vi "Main.vi"() -> ()   [LabVIEW 2021]
doc: "The myRIO Project template acquires acceleration data from the onboard accelerometer and displays the changes of acceleration values in a waveform chart."
uses:
  <vilib>/myRIO/Instrument Drivers/Onboard IO/AI/typedefs/AI Reference.ctl
  <vilib>/myRIO/Common/Instrument Driver Framework/Utilities/typedefs/myRIO Generic Hardware Reference.ctl
  <vilib>/myRIO/Common/Instrument Driver Framework/Utilities/typedefs/Hardware Version Enum.ctl
  <vilib>/myRIO/Common/Instrument Driver Framework/Utilities/typedefs/myRIO v1.0 Reference.ctl
  <vilib>/myRIO/Common/Instrument Driver Framework/Utilities/typedefs/Generic FPGA Reference.ctl
  <vilib>/myRIO/Common/Instrument Driver Framework/myRIO v1.0/AI/typedefs/AI Channels List.ctl
  <vilib>/myRIO/Common/Instrument Driver Framework/myRIO v1.0/AI/typedefs/AI Channels Enum.ctl
  <vilib>/myRIO/Common/Instrument Driver Framework/Utilities/typedefs/Analog Scaling Constants List.ctl
  <vilib>/myRIO/Common/Instrument Driver Framework/Utilities/typedefs/Analog Scaling Constants.ctl
  <vilib>/userDefined/High Color/nirio_resource_hc.ctl
  <vilib>/myRIO/Instrument Drivers/Onboard IO/DIO/typedefs/DIO Reference.ctl
  <vilib>/myRIO/Common/Instrument Driver Framework/myRIO v1.0/DIO/typedefs/DIO Channels List.ctl
  <vilib>/myRIO/Common/Instrument Driver Framework/myRIO v1.0/DIO/typedefs/DIO Channels Enum.ctl
  <vilib>/myRIO/Instrument Drivers/Onboard IO/PWM/typedefs/PWM Reference.ctl
  <vilib>/myRIO/Common/Instrument Driver Framework/myRIO v1.0/PWM/typedefs/PWM Channels Enum.ctl
  <vilib>/myRIO/Instrument Drivers/Onboard IO/PWM/typedefs/PWM Configuration.ctl
  <vilib>/myRIO/Common/Instrument Driver Framework/Utilities/vis/Is FPGA Ref Available.vi
  <vilib>/myRIO/Common/Instrument Driver Framework/myRIO v1.0/AI/vis/myRIO v1.1 Open AI.vi
  <vilib>/myRIO/Instrument Drivers/Onboard IO/AI/vis/Read.vi
  <vilib>/myRIO/Common/Instrument Driver Framework/myRIO v1.0/DIO/vis/myRIO v1.1 Open DIO.vi
  <vilib>/myRIO/Instrument Drivers/Onboard IO/DIO/vis/Write.vi
  <vilib>/myRIO/Common/Instrument Driver Framework/myRIO v1.0/PWM/vis/myRIO v1.1 Open PWM.vi
  <vilib>/myRIO/Instrument Drivers/Onboard IO/PWM/vis/Set Duty Cycle and Frequency.vi
  <vilib>/myRIO/Common/Instrument Driver Framework/Utilities/vis/Validate Channels.vi
  <vilib>/myRIO/Common/Instrument Driver Framework/myRIO v1.0/AI/vis/myRIO v1.0 Reserve AI.vi
  <vilib>/myRIO/Common/Instrument Driver Framework/myRIO v1.0/DIO/vis/myRIO v1.0 Reserve DIO.vi
  <vilib>/myRIO/Common/Instrument Driver Framework/myRIO v1.0/PWM/vis/myRIO v1.0 Reserve PWM.vi
  <vilib>/myRIO/Common/Instrument Driver Framework/myRIO v1.0/AI/vis/myRIO v1.0 Build MUX Configuration AI.vi
  <vilib>/myRIO/Common/Instrument Driver Framework/myRIO v1.0/Resource Manager/vis/myRIO v1.0 Reserve Channel List.vi
  <vilib>/myRIO/Common/Instrument Driver Framework/myRIO v1.0/DIO/vis/myRIO v1.0 Build MUX Configuration DIO.vi
  <vilib>/myRIO/Common/Instrument Driver Framework/myRIO v1.0/PWM/vis/myRIO v1.0 Build MUX Configuration PWM.vi
  <vilib>/myRIO/Common/Instrument Driver Framework/myRIO v1.0/Resource Manager/vis/myRIO v1.0 Reserve Channel.vi
  <vilib>/myRIO/Common/Instrument Driver Framework/myRIO v1.0/Resource Manager/vis/myRIO v1.0 Unreserve Channel.vi
  <vilib>/myRIO/Common/Instrument Driver Framework/myRIO v1.0/Resource Manager/vis/myRIO v1.0 Create Configuration List.vi
  <vilib>/myRIO/Common/Instrument Driver Framework/myRIO v1.0/Resource Manager/vis/myRIO v1.0 Build Mutex Name.vi
  <vilib>/Utility/VariantDataType/GetNumericInfo.vi
  <vilib>/Utility/error.llb/Error Cluster From Error Code.vi
  <vilib>/myRIO/Common/Instrument Driver Framework/myRIO v1.0/myRIO v1.1 Open.vi
  <vilib>/myRIO/Common/Instrument Driver Framework/myRIO v1.0/AI/vis/myRIO v1.0 Get Scaling Constants AI.vi
  <vilib>/myRIO/Common/Instrument Driver Framework/Utilities/vis/IO Manager.vi
  <vilib>/myRIO/Common/Instrument Driver Framework/Utilities/vis/Configuration Manager.vi
  <vilib>/myRIO/Common/Instrument Driver Framework/myRIO v1.0/myRIO v1.0 Close.vi
  <vilib>/myRIO/Common/Instrument Driver Framework/myRIO v1.0/AI/vis/myRIO v1.0 Read AI.vi
  <vilib>/myRIO/Common/Instrument Driver Framework/myRIO v1.0/Resource Manager/vis/myRIO v1.0 Configure IO.vi
  <vilib>/myRIO/Common/Instrument Driver Framework/myRIO v1.0/DIO/vis/myRIO v1.0 Write DIO.vi
  <vilib>/addons/control/pid/pid.llb/PID (DBL).vi
  <vilib>/myRIO/Common/Instrument Driver Framework/myRIO v1.0/PWM/vis/myRIO v1.0 Write PWM.vi
  <vilib>/myRIO/Express VI/Onboard IO/AI/AI Express VI.xnode
  <vilib>/myRIO/Instrument Drivers/Onboard IO/AI/vis/myRIO AI Open.xnode
  <vilib>/myRIO/Express VI/Onboard IO/DO/DO Express VI.xnode
  <vilib>/myRIO/Instrument Drivers/Onboard IO/DIO/vis/myRIO DIO Open.xnode
  <vilib>/myRIO/Express VI/Onboard IO/PWM/PWM Express VI.xnode
  <vilib>/myRIO/Instrument Drivers/Onboard IO/PWM/vis/myRIO PWM Open.xnode
  <vilib>/myRIO/Instrument Drivers/Onboard IO/AI/AI.lvlib
  <vilib>/myRIO/Instrument Drivers/Onboard IO/DIO/DIO.lvlib
  <vilib>/addons/control/pid/NI_PID_pid.lvlib
  <vilib>/myRIO/Instrument Drivers/Onboard IO/PWM/PWM.lvlib
panel:
  out "Array Index":dbl
  out "Target Angle Reached":bool
  in  "Drop-Off Angle":dbl=90.0
  in  "Complete Stop Angle":dbl=45.0
  out "Target Angle":dbl
  out "Drop-Off Position":dbl
  out "Complete Stop Position":dbl
  in  "PID Gains":T1={"Proportional Gain, Kc"=0.5, "Integral Time, ti"=0.1, "Derivative Time, td"=0.1}
  out "Run Motor PWM":dbl
  in  "Manual Mode switch":bool
  in  "DIO4":bool
  in  "DIO5":bool
  in  "DIO6":bool
  in  "DIO7":bool
  out "Upper limit":bool
  out "Lower Limit":bool
  in  "Home Position":dbl=250.0
  out "Angle":dbl
  out "AI3":dbl
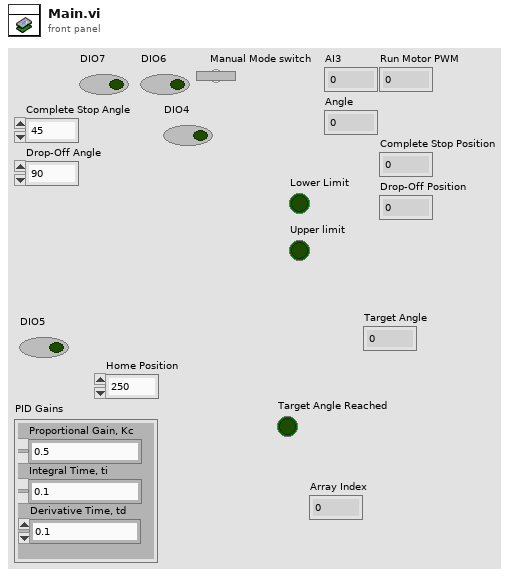
[diagram p1: front panel]
types:
  T1 = cluster{"Proportional Gain, Kc":dbl, "Integral Time, ti":dbl, "Derivative Time, td":dbl}
  T2 = typedef "DIO.lvlib/DIO Reference.ctl" = cluster{"myRIO Reference":T3, "DIO Channels List":T7}
  T3 = typedef "myRIO Generic Hardware Reference.ctl" = cluster{"myRIO Model":T4, "myRIO Hardware Reference":T5}
  T4 = typedef "Hardware Version Enum.ctl" = enum16{"Unknown", "myRIO-1900", "myRIO-1950", "roboRIO", "NI ELVIS RIO CM", "ELVIS III"}
  T5 = typedef "myRIO v1.0 Reference.ctl" = cluster{"Generic FPGA Reference":T6, "Allow multiple opens":bool}
  T6 = typedef "Generic FPGA Reference.ctl" = refnum<k20>
  T7 = typedef "DIO Channels List.ctl" = T8[]
  T8 = typedef "DIO Channels Enum.ctl" = enum16{"Not Connected", "C/DIO0", "C/DIO1", "C/DIO2", "C/DIO3", "C/DIO4", "C/DIO5", "C/DIO6", "C/DIO7", "A/DIO0", "A/DIO1", "A/DIO2", "A/DIO3", "A/DIO4", "A/DIO5", "A/DIO6", "A/DIO7", "A/DIO8", "A/DIO9", "A/DIO10", "A/DIO11", "A/DIO12", "A/DIO13", "A/DIO14", "A/DIO15", "A/DIO16", "A/DIO17", "A/DIO18", "A/DIO19", "B/DIO0", "B/DIO1", "B/DIO2", "B/DIO3", "B/DIO4", "B/DIO5", "B/DIO6", "B/DIO7", "B/DIO8", "B/DIO9", "B/DIO10", "B/DIO11", "B/DIO12", "B/DIO13", "B/DIO14", "B/DIO15", "B/DIO16", "B/DIO17", "B/DIO18", "B/DIO19", "LED0", "LED1", "LED2", "LED3", "Button0", "DIO/DIO0", "DIO/DIO1", "DIO/DIO2", "DIO/DIO3", "DIO/DIO4", "DIO/DIO5", "DIO/DIO6", "DIO/DIO7", "DIO/DIO8", "DIO/DIO9", "SPI/CS0", "SPI/CS1", "SPI/CS2", "SPI/CS3", "LED RADIO (Green)", "LED RADIO (Red)", "LED COMM (Green)", "LED COMM (Red)", "LED MODE (Green)", "LED MODE (Red)"}
  T9 = typedef "nirio_resource_hc.ctl" = tag
  T10 = typedef "PWM.lvlib/PWM Reference.ctl" = cluster{"myRIO Reference":T3, "PWM Channels Enum":T11, "PWM Configuration":T12}
  T11 = typedef "PWM Channels Enum.ctl" = enum16{"Not Connected", "C/PWM0", "C/PWM1", "A/PWM0", "A/PWM1", "A/PWM2", "A/PWM3", "A/PWM4", "A/PWM5", "A/PWM6", "A/PWM7", "A/PWM8", "A/PWM9", "A/PWM10", "A/PWM11", "A/PWM12", "A/PWM13", "A/PWM14", "A/PWM15", "A/PWM16", "A/PWM17", "A/PWM18", "A/PWM19", "B/PWM0", "B/PWM1", "B/PWM2", "B/PWM3", "B/PWM4", "B/PWM5", "B/PWM6", "B/PWM7", "B/PWM8", "B/PWM9", "B/PWM10", "B/PWM11", "B/PWM12", "B/PWM13", "B/PWM14", "B/PWM15", "B/PWM16", "B/PWM17", "B/PWM18", "B/PWM19", "PWM/PWM0", "PWM/PWM1", "PWM/PWM2", "PWM/PWM3", "PWM/PWM4", "PWM/PWM5", "PWM/PWM6", "PWM/PWM7", "PWM/PWM8", "PWM/PWM9"}
  T12 = typedef "PWM.lvlib/PWM Configuration.ctl" = cluster{"Frequency":dbl, "Duty Cycle":dbl}
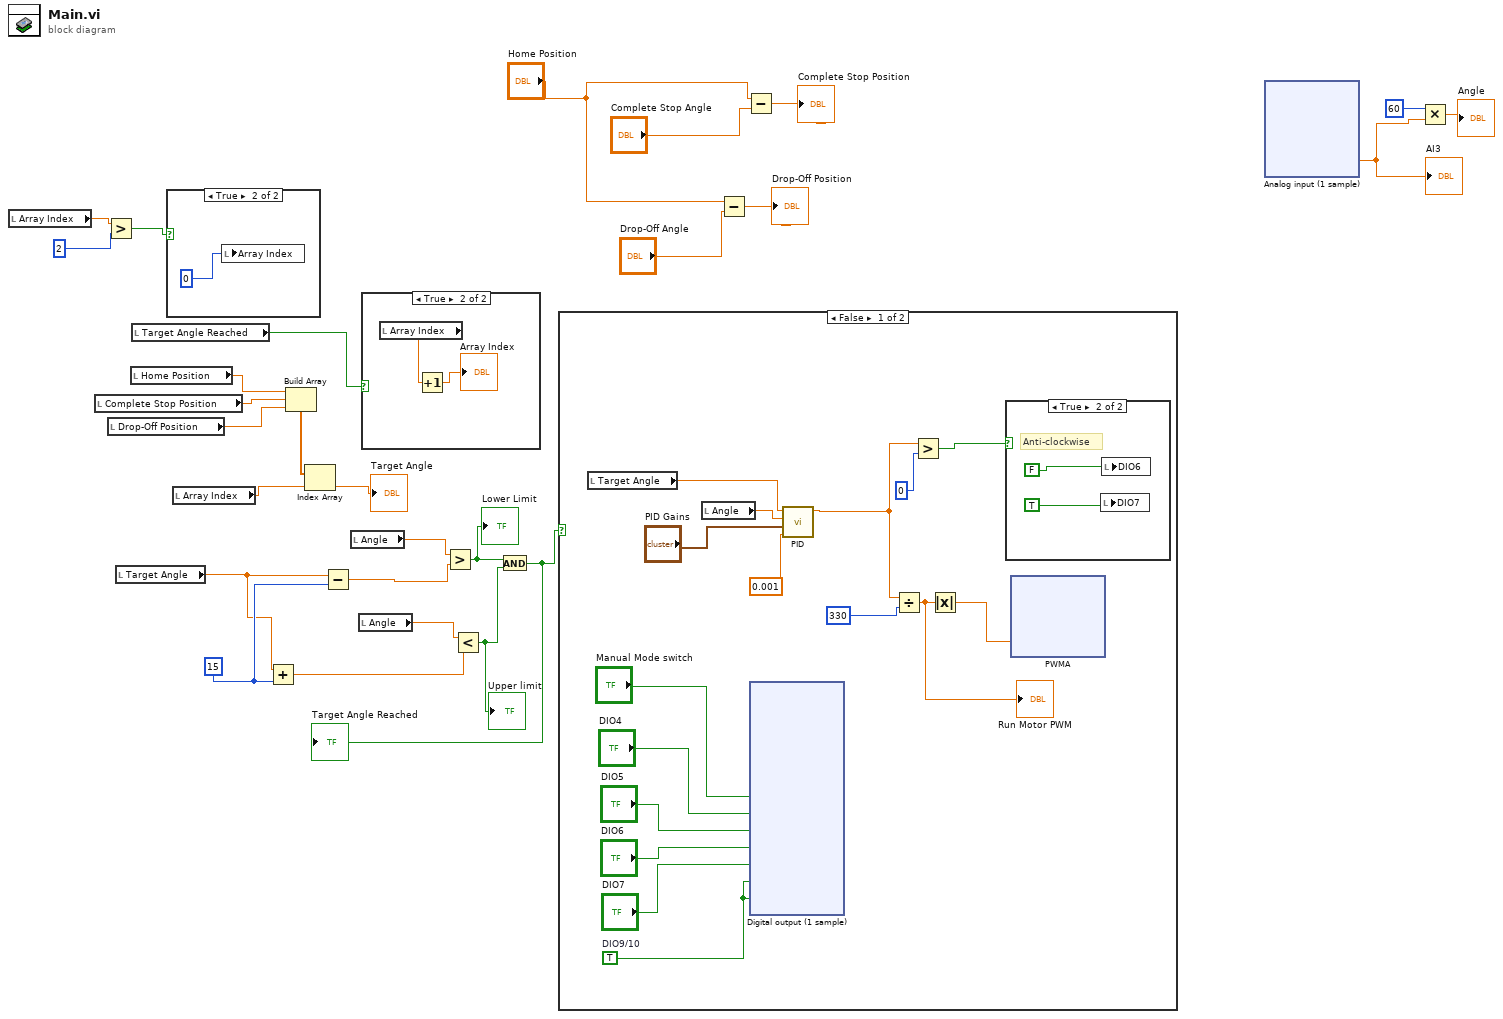
[diagram p0: block diagram]
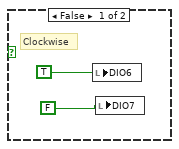
[diagram p4: hidden frame]
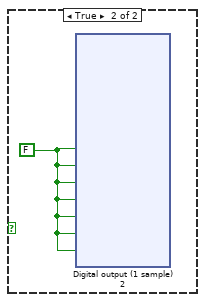
[diagram p5: hidden frame]
diagram:
  w18 = 15
  n1 = local read "Array Index"() -> (w2:dbl)
  n2 = local read "Complete Stop Position"() -> (w10:dbl)
  n3 = Greater?(x=w2, y=2) -> (0:w3:bool)
  n4 = local read "Drop-Off Position"() -> (w9:dbl)
  n5 = local read "Target Angle"() -> (w12:dbl)
  n6 = local read "Home Position"() -> (w11:dbl)
  n7 = local read "Target Angle Reached"() -> (w7:bool)
  n8 = case shown="True" w3 {
    frame False {
    }
    frame True {
      n9 = local write "Array Index"(0) -> ()
    }
  }
  n10 = local read "Array Index"() -> (w4:dbl)
  n11 = Add(x=w12, y=w18) -> (x+y=w20:dbl)
  n12 = Build Array(w11, w10, w9) -> (w5:dbl[])
  n13 = Index Array(array=w5, index=w4) -> (element=→"Target Angle":dbl)
  n14 = Subtract(x=w12, y=w18) -> (x-y=w19:dbl)
  n15 = local read "Angle"() -> (w24:dbl)
  n16 = local read "Angle"() -> (w23:dbl)
  n17 = case shown="True" w7 {
    frame False {
    }
    frame True {
      n18 = local read "Array Index"() -> (w29:dbl)
      n19 = Increment(x=w29) -> (x+1=→"Array Index":dbl)
    }
  }
  n20 = Greater?(x=w24, y=w19) -> (0:w22:bool)
  "Lower Limit" <- w22
  n21 = Less?(x=w23, y=w20) -> (x < y?=w21:bool)
  "Upper limit" <- w21
  n22 = And(x=w22, y=w21) -> (x .and. y?=w8:bool)
  "Target Angle Reached" <- w8
  n23 = case shown="False" w8 {
    frame False {
      w32 = TRUE  # DIO9/10
      n24 = local read "Target Angle"() -> (w31:dbl)
      n25 = local read "Angle"() -> (w46:dbl)
      n26 = xnode "Digital output (1 sample)"("Auto/Manual Mode Switch (A/DIO3 (Pin 17))"="Manual Mode switch", "Solenoid 1 (A/DIO4 (Pin 19))"="DIO4", "Solenoid 2 (A/DIO5 (Pin 21))"="DIO5", "Motor Clockwise (A/DIO6 (Pin 23))"="DIO6", "Motor Anti-Clockwise (A/DIO7 (Pin 25))"="DIO7", "Solenoid PWM (A/DIO9 (Pin 29))"=w32, "Motor Driver Chip Standby (A/DIO10 (Pin 31))"=w32) -> ()  [unwired: 1 in, 1 out]
      n27 = call-poly <vilib>:"PID.vi"("dt (s)"=0.001, "PID gains"="PID Gains", "process variable"=w46, "setpoint"=w31) -> ("output"=w42:dbl)  [unwired: 6 in, 1 out]
      n28 = Divide(x=w42, y=330) -> (x/y=w39:dbl)
      "Run Motor PWM" <- w39
      n29 = Greater?(x=w42, y=0) -> (0:w38:bool)
      n30 = Absolute Value(x=w39) -> (abs(x)=w41:dbl)
      n31 = case shown="True" w38 {
        frame False {
          # "Clockwise"
          n32 = local write "DIO6"(TRUE) -> ()
          n33 = local write "DIO7"(FALSE) -> ()
        }
        frame True {
          # "Anti-clockwise"
          n34 = local write "DIO7"(TRUE) -> ()
          n35 = local write "DIO6"(FALSE) -> ()
        }
      }
      n36 = xnode "PWMA"("Duty Cycle"=w41) -> ()  [unwired: 1 in, 1 out]
    }
    frame True {
      w127 = FALSE
      n37 = xnode "Digital output (1 sample) 2"("Auto/Manual Mode Switch (A/DIO3 (Pin 17))"=w127, "Solenoid 1 (A/DIO4 (Pin 19))"=w127, "Solenoid 2 (A/DIO5 (Pin 21))"=w127, "Motor Clockwise (A/DIO6 (Pin 23))"=w127, "Motor Anti-Clockwise (A/DIO7 (Pin 25))"=w127, "Solenoid PWM (A/DIO9 (Pin 29))"=w127, "Motor Driver Chip Standby (A/DIO10 (Pin 31))"=w127) -> ()  [unwired: 1 in, 1 out]
    }
  }
  n38 = Subtract(x="Home Position", y="Drop-Off Angle") -> (x-y=→"Drop-Off Position":dbl)
  n39 = Subtract(x="Home Position", y="Complete Stop Angle") -> (x-y=→"Complete Stop Position":dbl)
  n40 = xnode "Analog input (1 sample)"() -> ("Motor Position (A/AI3 (Pin 9))"=w25:dbl)  [unwired: 1 in, 1 out]
  "AI3" <- w25
  n41 = Multiply(x=60, y=w25) -> (x*y=→"Angle":dbl)
